vi "Geometric Matching.vi"() -> ()   [LabVIEW 2014]
doc: "This example shows how to use the geometric matching tools in NI Vision.\n\nGeometric matching is the technique used to quickly locate known reference or fiducial patterns in an image using edge information. Geometric matching is the key to many applications. Geometric matching can provide your application with information about the presence or absence, number, and location of the model within an image.\n\nAn important step in geometric matching is training the template. A specialized geometric training interface is provided for simple training with advanced features. This utility can be found at Start»Programs»National Instruments»Vision, or from Vision Assistant or Vision Builder for Automated Inspection."
uses:
  <vilib>/vision/NI_Vision_Development_Module.lvlib
panel:
  out "Results":string[][](table)
  in  "Minimum Score":sgl=800.0
  in  "Number of Matches":i32=4
  out "Template":T1(plugin-control)
  out "Number of Matches Found":i32
  in  "Stop":bool
  in  "Delay (s.)":dbl(slide)=0.496 scale=0.0..2.0
  out "Image":T1(plugin-control)
  # "Overview: Demonstrates how to use geometric matching to locate parts in an image.\nRequirements: NI Vision Development Module\nInstructions: Run the VI."
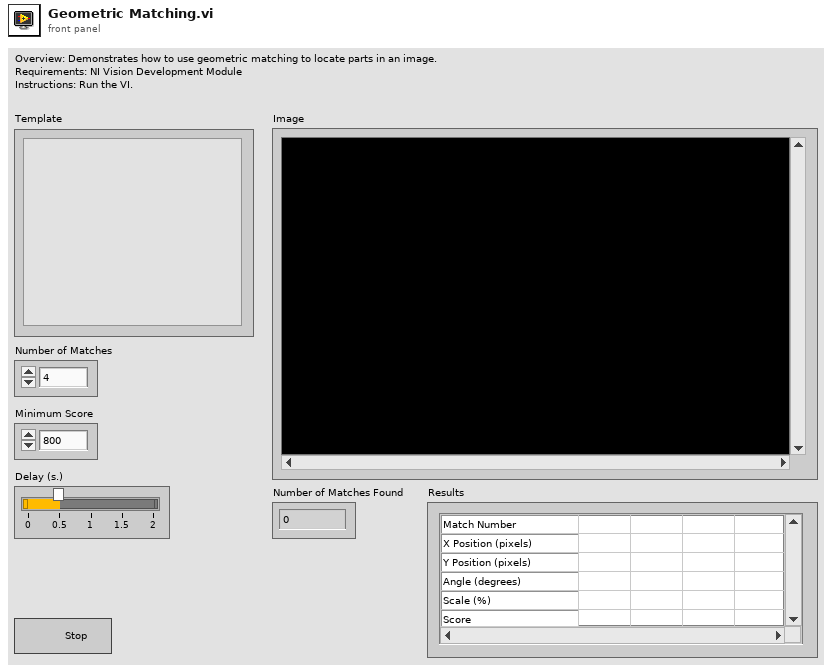
[diagram p1: front panel]
types:
  T1 = typedef "IMAQ Image.ctl" = refnum<image>
  T2 = typedef "Image Type" = u32
  T3 = cluster{"Rotation":bool, "Scale":bool, "Occlusion":bool, "Reserved":bool, "Reserved":bool, "Reserved":bool}
  T4 = typedef "IMAQ GM Match Report.ctl" = cluster{"Position":cluster{"x":sgl, "y":sgl}, "Angle":sgl, "Scale":sgl, "Score":sgl, "Bounding Box":cluster{"x":sgl, "y":sgl}[], "Contrast Reversed":bool, "Occlusion %":sgl, "Template Target Curve Score":sgl, "Target Template Curve Score":sgl, "Correlation Score":sgl}
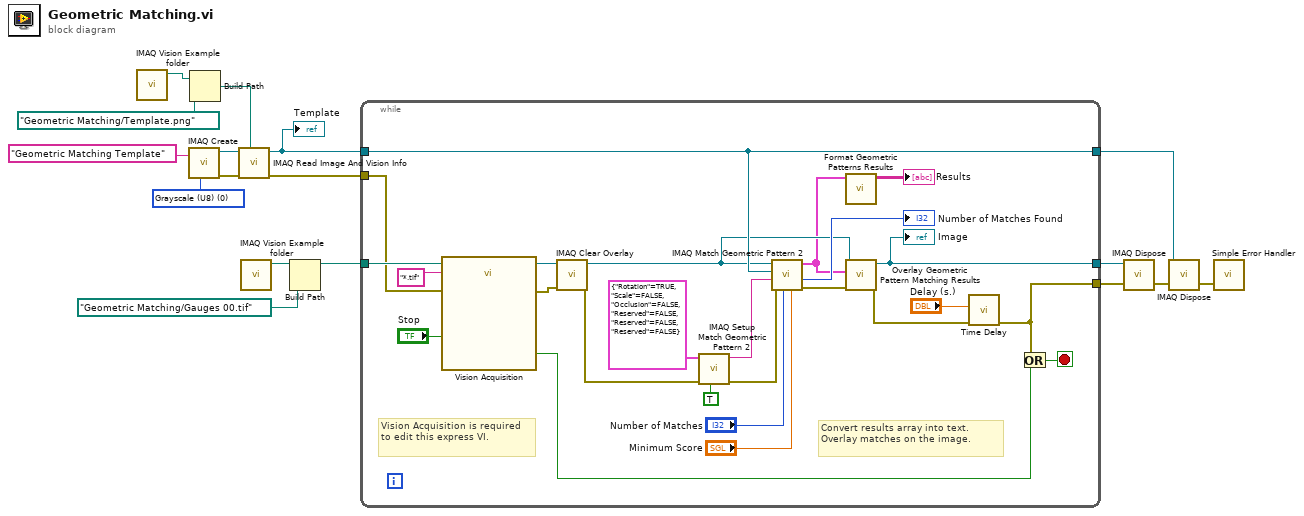
[diagram p0: block diagram]
diagram:
  w9 = T2 0 items=["Grayscale (U8)", "Grayscale (I16)", "Grayscale (SGL)", "Complex (CSG)", "RGB (U32)", "HSL (U32)", "RGB (U64)"] ("Image Type")
  n1 = call "IMAQ Vision Example folder.vi"() -> ("Example Image Path"=w7:path)  [unwired: 11 in]
  n2 = call "IMAQ Create"("Image Name"="Geometric Matching Template", "Image Type"=w9) -> ("New Image"=w10:T1, "error out"=w11:errorcluster)  [unwired: 2 in, 1 out]
  n3 = Build Path(base path=w7, name or relative path=path "Geometric Matching/Template.png") -> (appended path=w13:path)
  n4 = call "IMAQ Read Image And Vision Info"("File Path"=w13, "error in (no error)"=w11, "Image"=w10) -> ("error out"=w1:errorcluster, "Image Out"=w6:T1)  [unwired: 1 in, 6 out]
  "Template" <- w6
  n5 = call "IMAQ Vision Example folder.vi"() -> ("Example Image Path"=w17:path)  [unwired: 11 in]
  n6 = Build Path(base path=w17, name or relative path=path "Geometric Matching/Gauges 00.tif") -> (appended path=w15:path)
  n7 = while {
    tunnel: w15 -> [w41]
    tunnel: [w37] -> w14
    tunnel: w6 -> [w24]
    tunnel: [w18] -> w5
    tunnel: [w24] -> w4
    tunnel: w1 -> [w22]
    stop <- w38 stop-if-true
    # "Vision Acquisition is required to edit this express VI."
    # "Convert results array into text.\nOverlay matches on the image."
    n8 = call "Vision Acquisition"("Image Path"=w41, "Image File Type (All Types)"="*.tif", "Stop (F)"="Stop", "error in"=w22) -> ("Image Out"=w36:T1, "Stopped"=w39:bool, "error out"=w40:errorcluster)  [unwired: 21 in]
    n9 = call "IMAQ Clear Overlay"("error in (no error)"=w40, "Image"=w36) -> ("error out"=w27:errorcluster, "Image Out"=w21:T1)  [unwired: 1 in, 7 out]
    n10 = call "IMAQ Setup Match Geometric Pattern 2"("Use Learn Curve Parameters"=TRUE, "error in (no error)"=w27, "Match Mode"=T3 {"Rotation"=TRUE, "Scale"=FALSE, "Occlusion"=FALSE, "Reserved"=FALSE, "Reserved"=FALSE, "Reserved"=FALSE}) -> ("error out"=w33:errorcluster, "Match Geometric Pattern 2 Setup Data"=w31:string)  [unwired: 3 in, 4 out]
    n11 = call "IMAQ Match Geometric Pattern 2"("Minimum Match Score"="Minimum Score", "Number of Matches Requested"="Number of Matches", "error in (no error)"=w33, "Match Geometric Pattern 2 Setup Data"=w31, "Template Image"=w24, "Image"=w21) -> ("error out"=w28:errorcluster, "Number of Matches"=→"Number of Matches Found":i32, "Matches (pixel)"=w20:T4[])  [unwired: 1 in, 2 out]
    n12 = call "Format Geometric Patterns Results.vi"("Matches"=w20) -> ("Text Results"=→"Results":string[][])  [unwired: 9 in, 1 out]
    n13 = call "Overlay Geometric Pattern Matching Results.vi"("error in"=w28, "Matches"=w20, "Image"=w21) -> ("error out"=w25:errorcluster, "Image Out"=w18:T1)  [unwired: 2 in, 5 out]
    "Image" <- w18
    n14 = call "Time Delay"("error in (no error)"=w25, "Delay Time (s)"="Delay (s.)") -> ("error out"=w37:errorcluster)  [unwired: 9 in]
    n15 = Or(x=w37, y=w39) -> (x .or. y?=w38:bool)
  }
  n16 = call "IMAQ Dispose"("Image"=w5, "error in (no error)"=w14) -> ("error out"=w3:errorcluster)  [unwired: 1 in, 3 out]
  n17 = call "IMAQ Dispose"("Image"=w4, "error in (no error)"=w3) -> ("error out"=w2:errorcluster)  [unwired: 1 in, 3 out]
  n18 = call <vilib>:"Simple Error Handler.vi"("error in (no error)"=w2) -> ()  [unwired: 4 in, 5 out]
